vi "Read 1 Swipe Direction.vi"(8 "Error In":errorcluster, 11 "Leap Handle":T3) -> (0 "Error Out":errorcluster, 1 "Gesture State":T1, 2 "Swipe Direction":T2, 3 "Leap Handle":T3)   [LabVIEW 2011, in "LVH-Leap.lvlib"]
uses:
  LVH-Leap.lvlib
  Private/Type Defs/Leap Handle.ctl
  C:/github/labviewhacker/LVH-Leap/LabVIEW/vi.lib/LabVIEW Hacker/Leap/Private/Libs/LeapCSharp.NET3.5.dll
  Private/Libs/LeapCSharp.NET3.5.dll
  Private/Type Defs/Swipe Direction.ctl
  Private/Type Defs/Gesture State.ctl
  Read N Swipes.vi
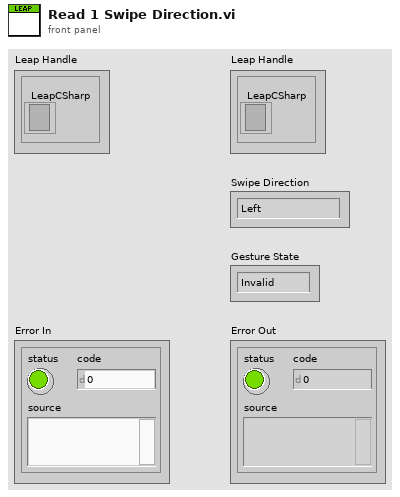
[diagram p1: front panel]
types:
  T1 = typedef "LVH-Leap.lvlib/Gesture State.ctl" = enum16{"Invalid", "Start", "Update", "Stop"}
  T2 = typedef "LVH-Leap.lvlib/Swipe Direction.ctl" = enum16{"Left", "Right", "Up", "Down", "In", "Out"}
  T3 = typedef "LVH-Leap.lvlib/Leap Handle.ctl" = cluster{"LeapCSharp":refnum<k24>}
  T4 = typedef "LVH-Leap.lvlib/Gesture Swipe.ctl" = cluster{"Common":T5, "Direction":T7, "Position":T7, "Start Position":T7, "Speed":dbl}
  T5 = typedef "LVH-Leap.lvlib/Gesture Common.ctl" = cluster{"ID":dbl, "Duration (S)":dbl, "Gesture Type":T6, "Gesture State":T1}
  T6 = typedef "LVH-Leap.lvlib/Gesture Type.ctl" = enum16{"Invalid", "Swipe", "Circle", "Screen Tap", "Key Tap"}
  T7 = typedef "LVH-Leap.lvlib/Vector.ctl" = cluster{"Pitch":sgl, "Yaw":sgl, "Roll":sgl, "Magnitude":sgl, "XYZ":sgl[]}
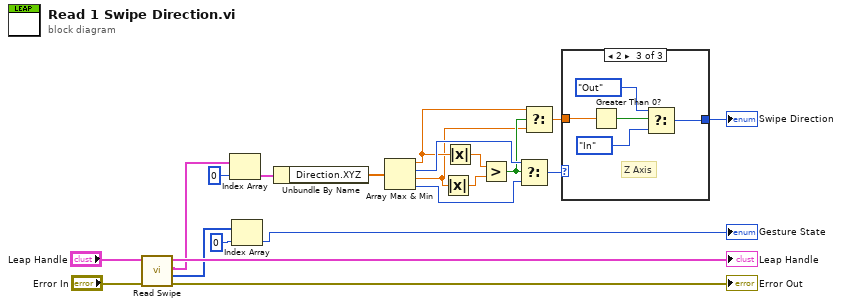
[diagram p0: block diagram]
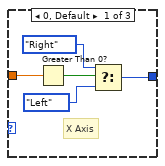
[diagram p2: hidden frame]
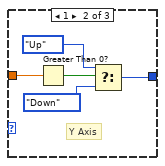
[diagram p3: hidden frame]
diagram:
  n1 = call-poly "Read Swipe.vi"("Error In"="Error In", "Leap Handle"="Leap Handle") -> ("Error Out"=→"Error Out":errorcluster, "Swipe Statuses"=w2:T1[], "Swipe Gestures"=w7:T4[], "Leap Handle"=→"Leap Handle":T3)  [unwired: 6 in]
  n2 = Index Array(array=w7, index=0) -> (element=w6:T4)
  n3 = Index Array(array=w2, index=0) -> (element=→"Gesture State":T1)
  n4 = Unbundle By Name(w6) -> ("Direction.XYZ"=w17:sgl[])
  n5 = Array Max & Min(array=w17) -> (max value=w10:sgl, max index (indices)=w14:i32, min value=w9:sgl, min index (indices)=w13:i32)
  n6 = Absolute Value(x=w9) -> (abs(x)=w15:sgl)
  n7 = Absolute Value(x=w10) -> (abs(x)=w16:sgl)
  n8 = Greater?(x=w16, y=w15) -> (0:w11:bool)
  n9 = Select(t=w14, s=w11, f=w13) -> (s? t:f=w12:i32)
  n10 = Select(t=w10, s=w11, f=w9) -> (s? t:f=w8:sgl)
  n11 = case shown="2" w12 {
    tunnel: w8 -> [w26 w31 w36]
    tunnel: [w22 w27 w32] -> w4
    frame 0, Default {
      # "X Axis"
      n12 = Greater Than 0?(x=w26) -> (x > 0?=w25:bool)
      n13 = Select(t=Swipe_Direction."Right" ("Swipe Direction"), s=w25, f=Swipe_Direction."Left" ("Swipe Direction")) -> (s? t:f=w22:T2)
    }
    frame 1 {
      # "Y Axis"
      n14 = Greater Than 0?(x=w31) -> (x > 0?=w30:bool)
      n15 = Select(t=Swipe_Direction."Up" ("Swipe Direction"), s=w30, f=Swipe_Direction."Down" ("Swipe Direction")) -> (s? t:f=w27:T2)
    }
    frame 2 {
      # "Z Axis"
      n16 = Greater Than 0?(x=w36) -> (x > 0?=w35:bool)
      n17 = Select(t=Swipe_Direction."Out" ("Swipe Direction"), s=w35, f=Swipe_Direction."In" ("Swipe Direction")) -> (s? t:f=w32:T2)
    }
  }
  "Swipe Direction" <- w4
